vi "pid_controller.vi"(0 "Motor Voltage 1 Sample Ago":dbl, 1 "Error 2 Samples Ago":dbl, 2 "Error 1 Sample Ago":dbl, 3 "Error (Current)":dbl, 11 "Time (dt)":dbl, 12 "Kp":dbl=0.10000000000000009 step=1.0, 13 "Ki":dbl step=2.0, 14 "Kd":dbl step=1.0) -> (15 "Motor Voltage for Next Sample":dbl)   [LabVIEW 2015]
panel:
  # "PID CONTROLLER VI"
  # "(USING BACKWARD APPROXIMATION)"
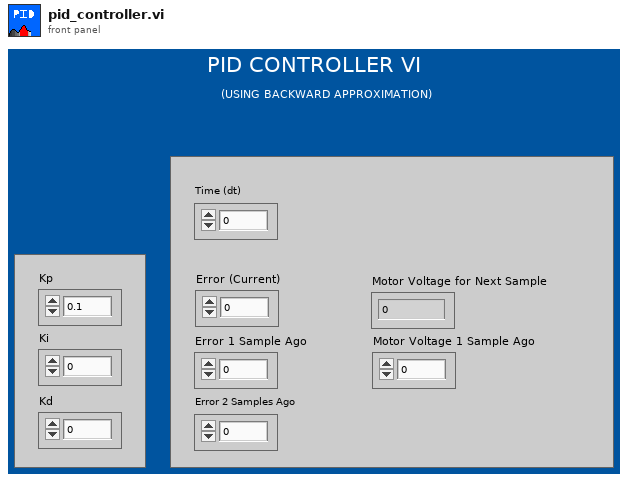
[diagram p1: front panel]
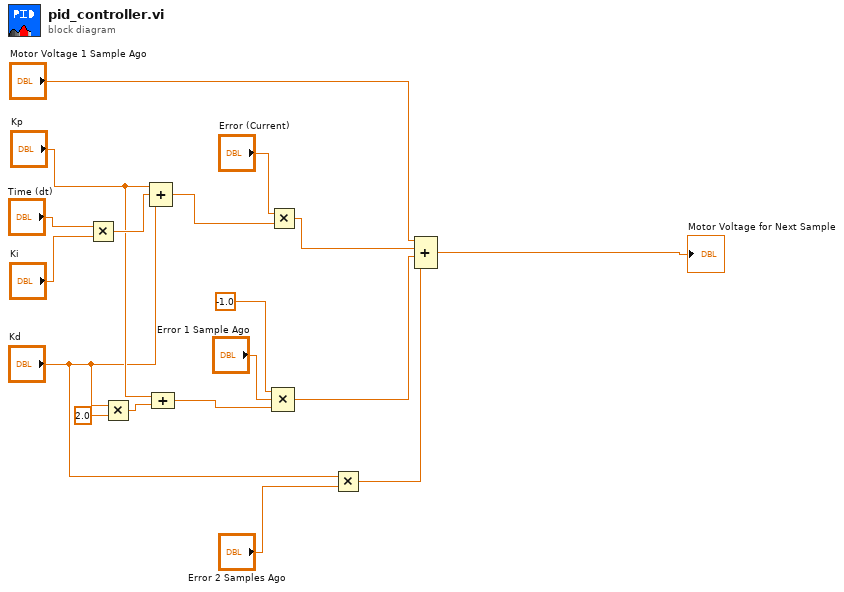
[diagram p0: block diagram]
diagram:
  n1 = Multiply(x="Time (dt)", y="Ki") -> (x*y=w13:dbl)
  n2 = Multiply(x="Kd", y=2.0) -> (x*y=w9:dbl)
  n3 = Compound Arithmetic op=ADD("Kp", w13, "Kd") -> (w12:dbl)
  n4 = Compound Arithmetic op=ADD("Kp", w9) -> (w5:dbl)
  n5 = Multiply(x="Error (Current)", y=w12) -> (x*y=w11:dbl)
  n6 = Compound Arithmetic op=MULTIPLY(-1.0 ("value"), "Error 1 Sample Ago", w5) -> (w4:dbl)
  n7 = Multiply(x="Kd", y="Error 2 Samples Ago") -> (x*y=w1:dbl)
  n8 = Compound Arithmetic op=ADD("Motor Voltage 1 Sample Ago", w11, w4, w1) -> (→"Motor Voltage for Next Sample":dbl)
